vi "Cleanup Events.vi"(8 "error in (no error)":errorcluster, 11 "Panel in":refnum<class "Panel.lvclass">) -> (0 "error out":errorcluster, 3 "Panel out":refnum<class "Panel.lvclass">)   [LabVIEW 2018, in "OOPanel.lvlib" / "Panel.lvclass"]
uses:
  Panel.lvclass
  Panel.lvclass/Panel.ctl
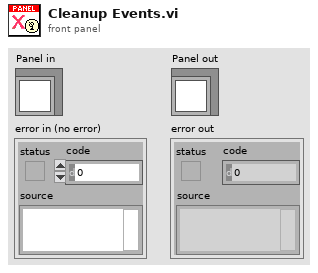
[diagram p1: front panel]
types:
  T1 = typedef "OOPanel.lvlib/Panel.lvclass/Ref Data.ctl" = cluster{"Panel VI":refnum<vi>, "Close":bool, "Panel Events":T2, "Running":bool, "Desired Size":T3, "Subpanel":refnum<vi>, "State":T4}
  T2 = typedef "OOPanel.lvlib/Panel.lvclass/Panel Events.ctl" = cluster{"Close":refnum<user-event>, "Visibility Changed":refnum<user-event>}
  T3 = typedef "OOPanel.lvlib/Panel.lvclass/Desired Size.ctl" = cluster{"Width":i16, "Height":i16}
  T4 = typedef "OOPanel.lvlib/Panel.lvclass/State.ctl" = enum16{"Idle", "Hidden", "Visible", "Subpanel"}
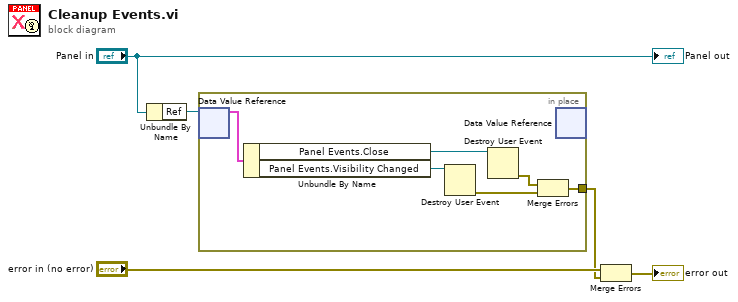
[diagram p0: block diagram]
diagram:
  n1 = Unbundle By Name("Panel in") -> ("Ref"=w4:refnum<data-value>)
  n2 = in-place {
    in-place-border: [w8] -> w1
    n3 = in-place-dvr #1(w4) -> (w11:T1)  [unwired: 1 out]
    n4 = Unbundle By Name(w11) -> ("Panel Events.Close"=w10:refnum<user-event>, "Panel Events.Visibility Changed"=w7:refnum<user-event>)
    n5 = Destroy User Event(user event=w7) -> (error out=w6:errorcluster)  [unwired: 1 in]
    n6 = Destroy User Event(user event=w10) -> (error out=w9:errorcluster)  [unwired: 1 in]
    n7 = Merge Errors(w9, w6) -> (w8:errorcluster)
    n8 = in-place-dvr #1() -> ()  [unwired: 1 in, 2 out]
  }
  n9 = Merge Errors("error in (no error)", w1) -> (→"error out":errorcluster)
  "Panel out" <- "Panel in"
